vi "Log.Record Main Queue Activity.vi"(7 "Level":T1=enum."Debug1" caption="Level(Normal)", 8 "Sub":string, 9 "Cmd":string, 10 "Module":string, 11 "LogIn":refnum<class "Event Notification.lvclass">) -> ()   [LabVIEW 2018]
uses:
  <vilib>/KATE/Event Log/Event Notification/Event Notification.lvclass
  <vilib>/KATE/Event Log/Event Notification/Event Log.Log Level.ctl
  <vilib>/KATE/Event Log/Event Log.lvlib
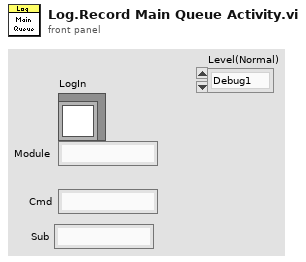
[diagram p1: front panel]
types:
  T1 = typedef "KATE_Lib.lvlib/Event Log.lvlib/Event Log.Log Level.ctl" = enum16{"Normal", "Verbose", "Debug0", "Debug1", "Debug2"}
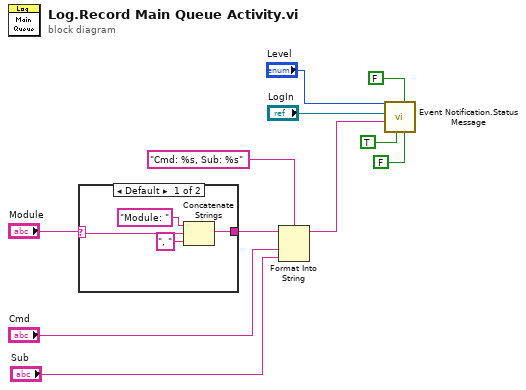
[diagram p0: block diagram]
diagram:
  n1 = case shown="Default" "Module" {
    selector: "Module" -> [w14 _]
    tunnel: [w13 _] -> w5
    frame Default {
      n2 = Concatenate Strings("Module: ", w14, ", " ("string")) -> (w13:string)
    }
    frame "" {
    }
  }
  n3 = Format Into String(format string="Cmd: %s, Sub: %s", initial string=w5, "Cmd", "Sub") -> (resulting string=w1:string)  [unwired: 1 in, 1 out]
  n4 = call <vilib>:"Event Notification.Status Message.vi"("Display"=FALSE, "FWD"=FALSE, "Log"=TRUE, "Level"="Level", "Message"=w1, "Event Notification in"="LogIn") -> ()  [unwired: 6 in]
